vi "svc_Coerce Index and Length.vi"(7 "input length":i32, 8 "error in (no error)":errorcluster, 10 "subset length (-1 = all)":i32, 11 "subset start index (0)":i32) -> (0 "error out":errorcluster, 2 "actual subset length":i32, 3 "actual start index":i32, 5 "end reached":bool)   [LabVIEW 2017]
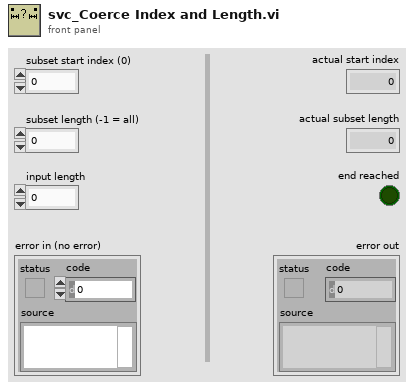
[diagram p1: front panel]
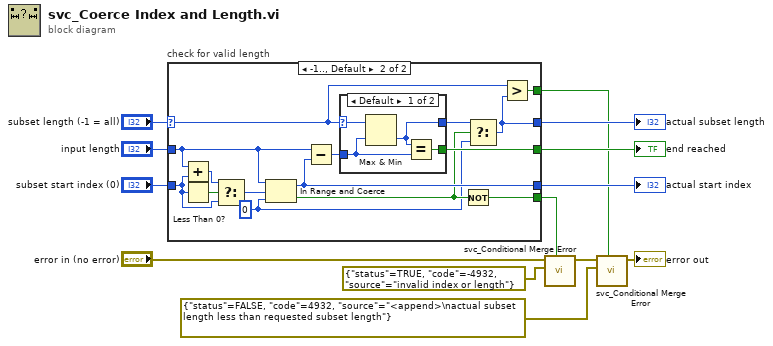
[diagram p0: block diagram]
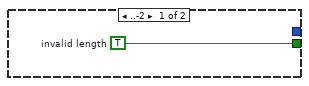
[diagram p2: hidden frame]
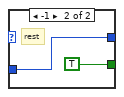
[diagram p3: hidden frame]
diagram:
  n1 = case "check for valid length" shown="-1.., Default" "subset length (-1 = all)" {
    selector: "subset length (-1 = all)" -> [_ w16]
    tunnel: "subset start index (0)" -> [_ w28]
    tunnel: [w14 w19] -> w7
    tunnel: "input length" -> [_ w22]
    tunnel: [_ w23] -> w12
    tunnel: [_ w17] -> w9
    tunnel: [_ w25] -> w13
    tunnel: [_ w15] -> w4
    frame ..-2 {
      w14 = TRUE  # invalid length
    }
    frame -1.., Default {
      w18 = 0 ("lower limit")
      n2 = Add(x=w22, y=w28) -> (x+y=w27:i32)
      n3 = Less Than 0?(x=w28) -> (x < 0?=w29:bool)
      n4 = Select(t=w27, s=w29, f=w28) -> (s? t:f=w24:i32)
      n5 = In Range and Coerce(upper limit=w22, x=w24, lower limit=w18) -> (coerced(x)=w23:i32, In Range?=w21:bool)
      n6 = Subtract(x=w22, y=w23) -> (x-y=w26:i32)
      n7 = case shown="Default" w16 {
        selector: w16 -> [w33 _]
        tunnel: [w32 w35] -> w20
        tunnel: w26 -> [w30 w35]
        tunnel: [w31 TRUE ("end reached")] -> w25
        frame Default {
          n8 = Max & Min(x=w33, y=w30) -> (min(x,y)=w32:i32)  [unwired: 1 out]
          n9 = Equal?(x=w32, y=w30) -> (x = y?=w31:bool)
        }
        frame -1 {
          # "rest"
        }
      }
      n10 = Not(x=w21) -> (.not. x?=w19:bool)
      n11 = Select(t=w20, s=w21, f=w18) -> (s? t:f=w17:i32)
      n12 = Greater?(x=w16, y=w17) -> (0:w15:bool)
    }
  }
  "end reached" <- w13
  "actual start index" <- w12
  "actual subset length" <- w9
  n13 = call <vilib>:"svc_Conditional Merge Error.vi"("merge"=w7, "new error"=errorcluster {"status"=TRUE, "code"=-4932, "source"="invalid index or length"} ("error out"), "error in (no error)"="error in (no error)") -> ("error out"=w2:errorcluster)  [unwired: 8 in]
  n14 = call <vilib>:"svc_Conditional Merge Error.vi"("merge"=w4, "new error"=errorcluster {"status"=FALSE, "code"=4932, "source"="<append>\nactual subset length less than requested subset length"} ("error out"), "error in (no error)"=w2) -> ("error out"=→"error out":errorcluster)  [unwired: 8 in]
